vi "FTW-Endpoint-CreateSender.vi"(0 "FTW Endpoint":refnum<class "FTW-Endpoint-TCP.lvclass">, 5 "Endpoint Address":string, 11 "error in":errorcluster) -> (4 "FTW Endpoint out":refnum<class "FTW-Endpoint-TCP.lvclass">, 15 "error out":errorcluster)   [LabVIEW 2013, in "FTW-Endpoint-TCP.lvclass"]
uses:
  FTW-Endpoint-TCP.lvclass
  Endpoint/FTW-Endpoint.lvclass
  FTW-Endpoint-TCP.lvclass/FTW-Endpoint-TCP.ctl
panel:
  # "Inputs"
  # "Outputs"
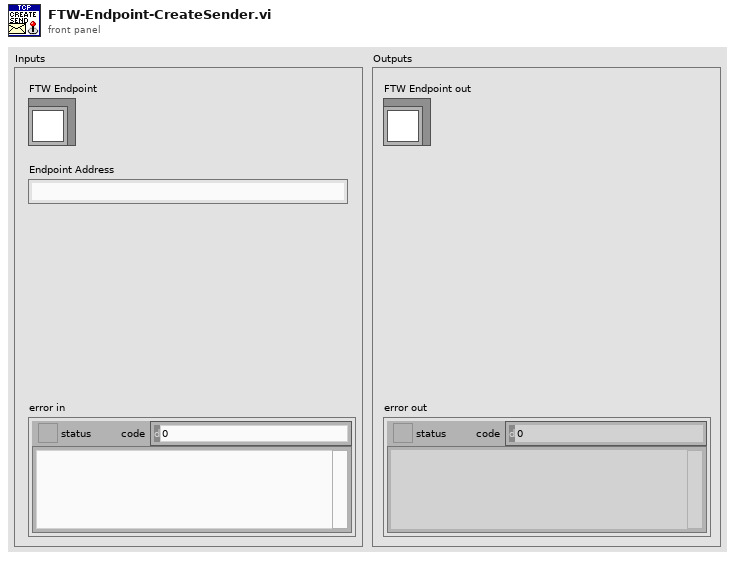
[diagram p1: front panel]
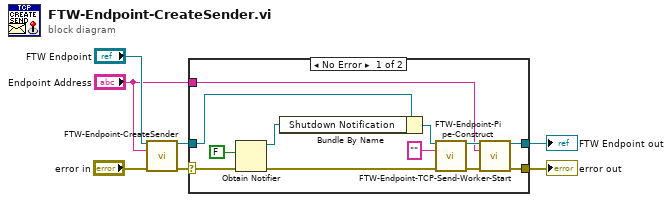
[diagram p0: block diagram]
diagram:
  n1 = call-parent "FTW-Endpoint-CreateSender.vi"("FTW Endpoint"="FTW Endpoint", "Endpoint Address"="Endpoint Address", "error in"="error in") -> ("FTW Endpoint out"=w6:refnum<class "FTW-Endpoint-TCP.lvclass">, "error out"=w4:errorcluster)  [unwired: 11 in]
  n2 = case shown="No Error" w4 {
    selector: w4 -> [w14 w20]
    tunnel: w6 -> [w13 w21]
    tunnel: [w15 w21] -> w3
    tunnel: [w17 w20] -> w2
    tunnel: "Endpoint Address" -> [w9 _]
    frame No Error {
      n3 = Obtain Notifier(notification data type=FALSE, error in (no error)=w14) -> (notifier out=w16:refnum<notifier>, error out=w18:errorcluster)  [unwired: 2 in, 1 out]
      n4 = Bundle By Name(cluster=w13, "Shutdown Notification"=w16) -> (w11:refnum<class "FTW-Endpoint-TCP.lvclass">)
      n5 = call-dynamic "FTW-Endpoint-Pipe-Construct.vi"("FTW Endpoint"=w11, "Address"="", "error in"=w18) -> ("FTW Endpoint out"=w10:refnum<class "FTW-Endpoint-TCP.lvclass">, "error out"=w12:errorcluster)  [unwired: 10 in, 1 out]
      n6 = call-dynamic "FTW-Endpoint-TCP-Send-Worker-Start.vi"("FTW-Endpoint-TCP In"=w10, "Endpoint Address"=w9, "error in"=w12) -> ("FTW-Endpoint-TCP Out"=w15:refnum<class "FTW-Endpoint-TCP.lvclass">, "error out"=w17:errorcluster)  [unwired: 11 in]
    }
    frame Error {
    }
  }
  "error out" <- w2
  "FTW Endpoint out" <- w3
